vi "Kicker_Collect_Kicking_Plate.vi"(8 "error in":errorcluster, 10 "Stop Position":dbl=3.4 format="%#_13g", 11 "Motor Speed":dbl=0.25) -> (0 "error out":errorcluster, 2 "Boolean":bool, 3 "Pot Position":dbl)   [LabVIEW 2017]
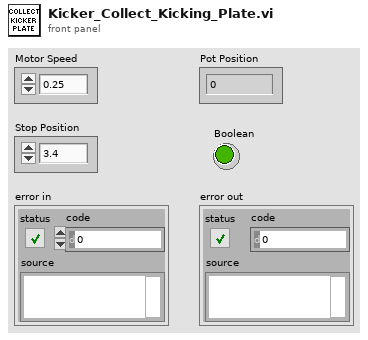
[diagram p1: front panel]
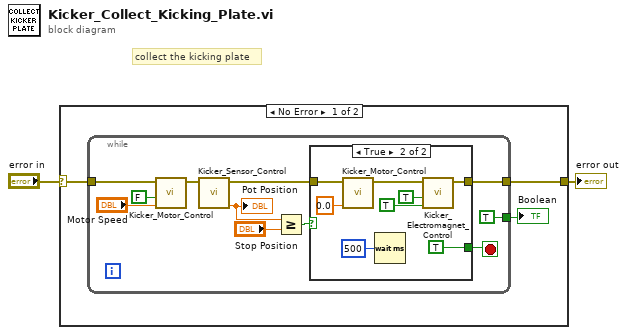
[diagram p0: block diagram]
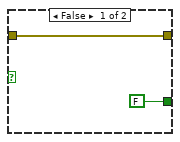
[diagram p2: hidden frame]
diagram:
  # "collect the kicking plate"
  n1 = case shown="No Error" "error in" {
    selector: "error in" -> [w4 w27]
    tunnel: [w5 w27] -> w2
    frame No Error {
      n2 = while {
        tunnel: [w7] -> w5
        tunnel: w4 -> [w11]
        tunnel: [TRUE] -> w3
        stop <- w16 stop-if-true
        n3 = call "Kicker_Motor_Control.vi"("Duty Cycle"="Motor Speed", "Motor Dir"=FALSE, "error in"=w11) -> ("error out"=w10:errorcluster)  [unwired: 8 in]
        n4 = call "Kicker_Sensor_Control.vi"("error in"=w10) -> ("Pot Output"=w9:dbl, "error out"=w8:errorcluster)  [unwired: 9 in]
        "Pot Position" <- w9
        n5 = Greater Or Equal?(x=w9, y="Stop Position") -> (x >= y?=w14:bool)
        n6 = case shown="True" w14 {
          tunnel: [FALSE TRUE] -> w16
          tunnel: w8 -> [w17 w20]
          tunnel: [w17 w19] -> w7
          frame False {
          }
          frame True {
            n7 = call "Kicker_Motor_Control.vi"("Duty Cycle"=0.0, "error in"=w20) -> ("error out"=w21:errorcluster)  [unwired: 9 in]
            n8 = Wait (ms)(milliseconds to wait=u32 500) -> ()  [unwired: 1 out]
            n9 = call "Kicker_Electromagnet_Control.vi"("Mag Enable"=TRUE, "Mag Dir"=TRUE, "error in"=w21) -> ("error out"=w19:errorcluster)  [unwired: 8 in]
          }
        }
      }
      "Boolean" <- w3
    }
    frame Error {
    }
  }
  "error out" <- w2
